vi "Convert I32 to SGL.vi"(9 "Input Valid":bool=TRUE, 10 "Input (I32)":i32) -> (1 "Output Valid":bool, 2 "Output (SGL)":sgl)   [LabVIEW 2014]
doc: "<b> Latency = 6 Ticks </b>"
panel:
  # "Copyright 2014 Vidrio Technologies\nScanImage 5 software is licensed under the Apache License, Version 2.0 (the \"License\"); you may not use any files contained\nwithin the ScanImage 5 release except in compliance with the License. You may obtain a copy of the License at\n http://www.apache.org/licenses/LICENSE-2.0\nUnless required by applicable law or agreed to in writing, software distributed under the License is distributed on an\n\"AS IS\" BASIS, WITHOUT WARRANTIES OR CONDITIONS OF ANY KIND, either express or implied. See the License for the\n specific language governing permissions and limitations under the License."
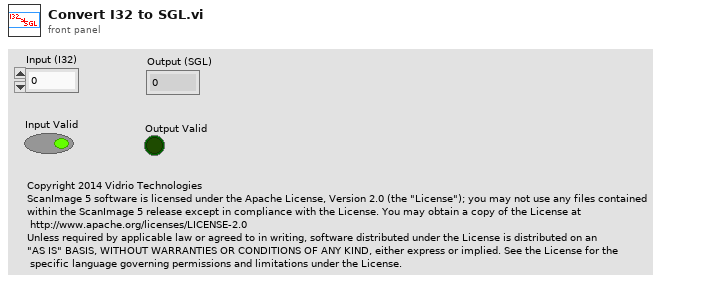
[diagram p1: front panel]
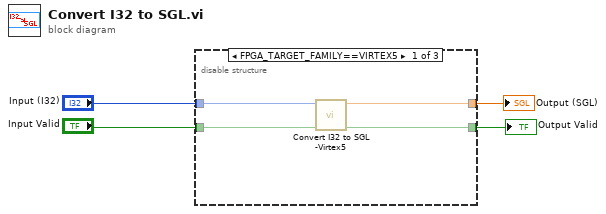
[diagram p0: block diagram]
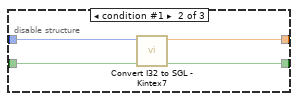
[diagram p2: hidden frame]
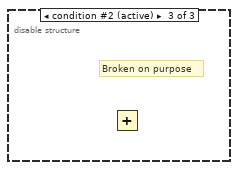
[diagram p3: hidden frame]
diagram:
  n1 = disable-structure shown="FPGA_TARGET_FAMILY==VIRTEX5" {
    disable-tunnel: "Input (I32)" -> [w8 w12 _]
    disable-tunnel: [w7 w11 _] -> w3
    disable-tunnel: "Input Valid" -> [w6 w10 _]
    disable-tunnel: [w5 w9 _] -> w1
    frame condition #0 {
      n2 = call "Convert I32 to SGL -Virtex5.vi"("Data In"=w8, "Data Valid In"=w6) -> ("Data Out"=w7:sgl, "Data Valid Out"=w5:bool)  [unwired: 7 in]
    }
    frame condition #1 {
      n3 = call "Convert I32 to SGL - Kintex7.vi"("Data In"=w12, "Data Valid In"=w10) -> ("Data Out"=w11:sgl, "Data Valid Out"=w9:bool)  [unwired: 7 in]
    }
    frame condition #2 (active) {
      # "Broken on purpose"
      n4 = Add() -> ()  [unwired: 2 in, 1 out]
    }
  }
  "Output (SGL)" <- w3
  "Output Valid" <- w1
